vi "Get File Folder Details.vi"(0 "Path":path, 11 "Error In":errorcluster) -> (4 "Parent Path":path, 6 "Name":string, 8 "Size":string, 15 "Error Out":errorcluster)   [LabVIEW 2023, in "File and Path Operations.lvlib"]
doc: "This VI accepts a file or folder path and returns the parent folder path, name and size."
uses:
  File and Path Operations.lvlib
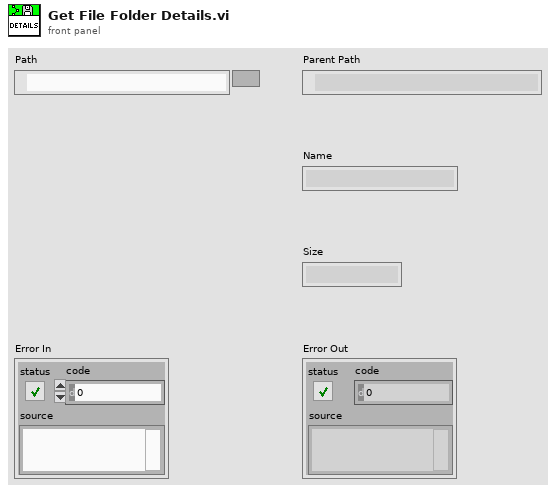
[diagram p1: front panel]
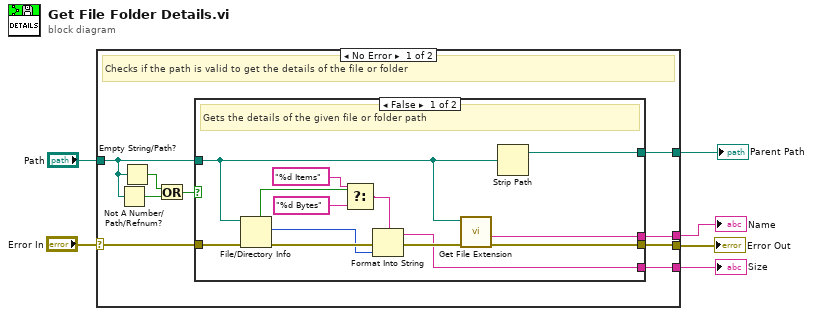
[diagram p0: block diagram]
diagram:
  n1 = case shown="No Error" "Error In" {
    selector: "Error In" -> [w15 w30]
    tunnel: [w14 w30] -> w5
    tunnel: [w12 _] -> w4
    tunnel: [w13 _] -> w3
    tunnel: [w11 _] -> w2
    tunnel: "Path" -> [w10 _]
    frame No Error {
      # "Checks if the path is valid to get the details of the file or folder"
      n2 = Not A Number/Path/Refnum?(number/path/refnum=w10) -> (NaN/Path/Refnum?=w8:bool)
      n3 = Empty String/Path?(string/path=w10) -> (empty?=w9:bool)
      n4 = Or(x=w9, y=w8) -> (x .or. y?=w7:bool)
      n5 = case shown="False" w7 {
        tunnel: w15 -> [w28 w29]
        tunnel: [w27 w29] -> w14
        tunnel: [w26 _] -> w13
        tunnel: [w23 _] -> w12
        tunnel: [w22 _] -> w11
        tunnel: w10 -> [w17 _]
        frame False {
          # "Gets the details of the given file or folder path"
          n6 = File/Directory Info(path=w17, error in=w28) -> (directory=w18:bool, size=w21:i64, error out=w25:errorcluster)  [unwired: 4 out]
          n7 = Select(t="%d Items" ("format string"), s=w18, f="%d Bytes") -> (s? t:f=w16:string)
          n8 = Format Into String(format string=w16, error in=w25, w21) -> (resulting string=w22:string, error out=w24:errorcluster)  [unwired: 1 in]
          n9 = call <vilib>:"Get File Extension.vi"("error in (no error)"=w24, "file"=w17) -> ("error out"=w27:errorcluster, "filename without extension"=w26:string)  [unwired: 5 in, 3 out]
          n10 = Strip Path(path=w17) -> (stripped path=w23:path)  [unwired: 1 out]
        }
        frame True {
        }
      }
    }
    frame Error {
      # "Return default values"
    }
  }
  "Name" <- w3
  "Parent Path" <- w4
  "Error Out" <- w5
  "Size" <- w2
